vi "_s_Cambio flujos manual.vi"(7 "Comunicaciones":T2={"Flujo_1"="ASRL6::INSTR", "Brk1"=FALSE, "Flujo_2"="ASRL6::INSTR", "Brk2"=FALSE, "Flujo_3"="ASRL6::INSTR", "Brk3"=FALSE, "Flujo_4"="ASRL6::INSTR", "Brk4"=FALSE, "Eurothe"="ASRL6::INSTR", "Eurot"=FALSE, "Balanza"="ASRL6::INSTR", "Bal"=FALSE, "eValPos"="ASRL6::INSTR", "eVal"=FALSE, "flowbus"="ASRL6::INSTR", "fb"=FALSE}, 8 "error in (no error)":errorcluster, 11 "Dispositivos":T3=[["3", "NO", "M0000013", "Air", "1", "ln/mn", "0", "0"], ["4", "NO", "M0000014", "Air", "1", "ln/mn", "0", "0"], ["5", "NO", "M0000015", "Air", "1", "ln/mn", "0", "0"], ["6", "NO", "M0000016", "Air", "1", "ln/mn", "0", "0"], ["7", "NO", "M0000017", "Air", "1", "ln/mn", "0", "0"], ["8", "NO", "M0000018", "Air", "1", "ln/mn", "0", "0"], ["9", "NO", "M0000019", "Air", "1", "ln/mn", "0", "0"], ["10", "NO", "M0000020", "Air", "1", "ln/mn", "0", "0"], ["11", "NO", "M0000021", "Air", "1", "ln/mn", "0", "0"]] caption="MassFlowControllers") -> (0 "error out":errorcluster, 1 "Setpoints":T1 {"SP4" format="%.2f"; "SP3" format="%.2f"; "SP2" format="%.2f"; "SP1" format="%.2f"})   [LabVIEW 2013]
doc: "Use this template to create a dialog box. This template polls the state of the buttons on the front panel and does not use events. Use the Dialog Using Events template (not available in Base package) to create a dialog box with event handling."
uses:
  _s_TablaBronkhorst.ctl
  Controles/P2018 Com Control.ctl
  Controles/P2019 SetpointsFlows.ctl
  _s_Bronkhorst Control.ctl
panel:
  out "SP4":dbl format="%.2f"
  out "SP3":dbl format="%.2f"
  out "SP2":dbl format="%.2f"
  in  "Salir":bool
  out "SP1":dbl format="%.2f"
  in  "Add 4":bool
  in  "Add 3":bool
  in  "Add 2":bool
  in  "Add 1":bool
  # "Nuevos flujos de gases (SERIE)"
  # "Setpoint"
  # "Nota: \nAl hacer CLICK en el pulsador aparecerá\nla ventana para establecer el nuevo setpoint"
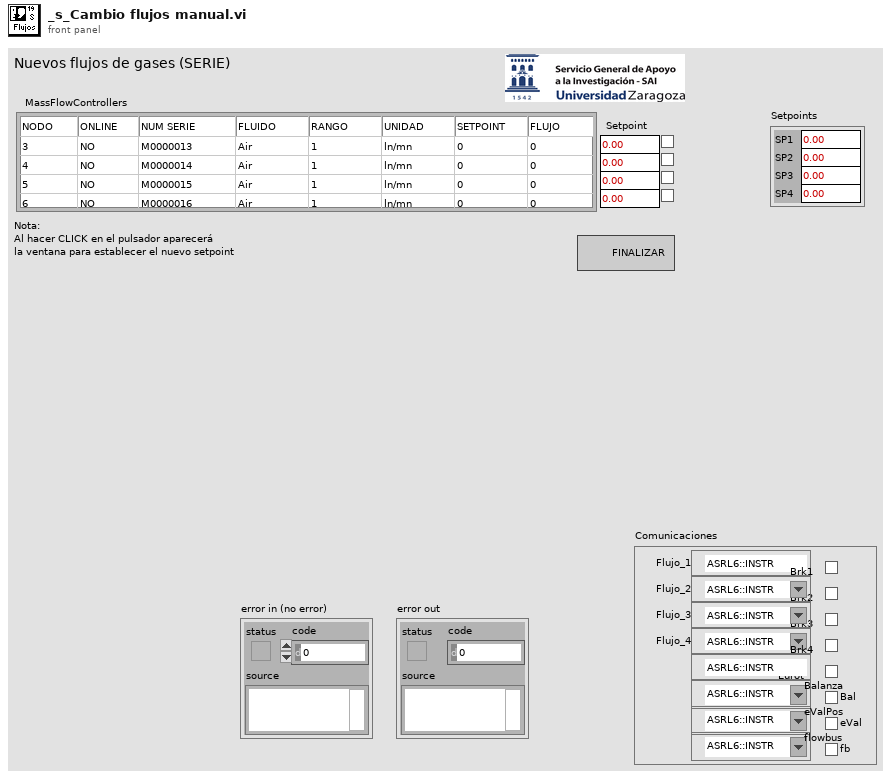
[diagram p1: front panel]
types:
  T1 = typedef "P2019 SetpointsFlows.ctl" = cluster{"SP1":dbl, "SP2":dbl, "SP3":dbl, "SP4":dbl}
  T2 = typedef "P2018 Com Control.ctl" = cluster{"Flujo_1":refnum<visa-resource-name>, "Brk1":bool, "Flujo_2":refnum<visa-resource-name>, "Brk2":bool, "Flujo_3":refnum<visa-resource-name>, "Brk3":bool, "Flujo_4":refnum<visa-resource-name>, "Brk4":bool, "Eurothe":refnum<visa-resource-name>, "Eurot":bool, "Balanza":refnum<visa-resource-name>, "Bal":bool, "eValPos":refnum<visa-resource-name>, "eVal":bool, "flowbus":refnum<visa-resource-name>, "fb":bool}
  T3 = typedef "_s_TablaBronkhorst.ctl" = string[][]
  T4 = typedef "_s_Bronkhorst Control.ctl" = enum16{"Inicializar", "Request IdnString", "Request Serial Number", "Request Fluid Number", "Request Fluid Name", "Request Sensor Type", "Request Cap 0", "Request Cap100", "Request Units", "Request CapUnitStr", "Request Setpoint %", "Request Setpoint", "Request Measure %", "Request Measure ", "Send Control Mode", "Send Fluid Number", "Send Setpoint %", "Send Setpoint", "Shutdown"}
  T5 = cluster{"SP1":dbl, "SP2":dbl, "SP3":dbl, "SP4":dbl}
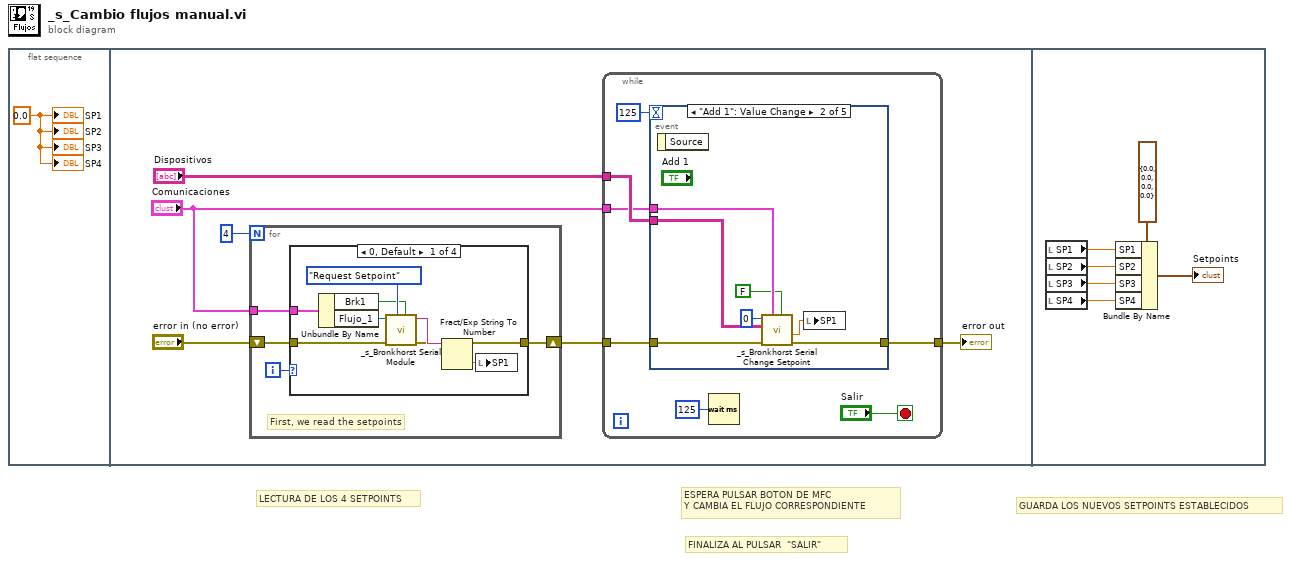
[diagram p0: block diagram]
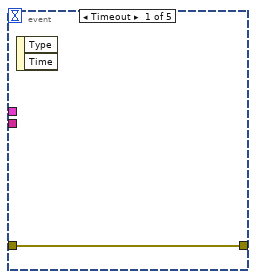
[diagram p2: hidden frame]
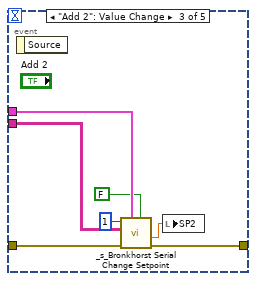
[diagram p3: hidden frame]
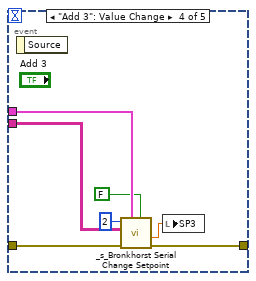
[diagram p4: hidden frame]
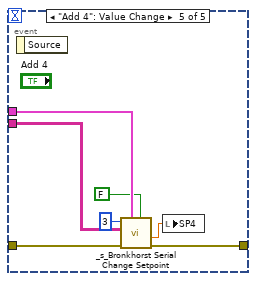
[diagram p5: hidden frame]
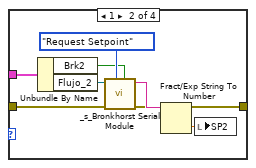
[diagram p6: hidden frame]
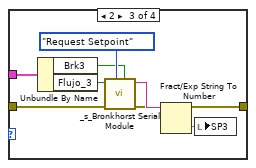
[diagram p7: hidden frame]
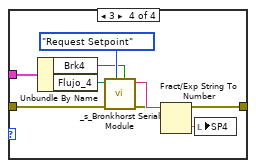
[diagram p8: hidden frame]
diagram:
  # "FINALIZA AL PULSAR  \"SALIR\""
  # "GUARDA LOS NUEVOS SETPOINTS ESTABLECIDOS"
  # "ESPERA PULSAR BOTON DE MFC\nY CAMBIA EL FLUJO CORRESPONDIENTE"
  # "LECTURA DE LOS 4 SETPOINTS"
  n1 = flat-sequence {
    frame #0 {
      w1 = 0.0 ("SP1")
      "SP1" <- w1
      "SP2" <- w1
      "SP3" <- w1
      "SP4" <- w1
    }
    frame #1 {
      n2 = for {
        N: 4 -> [_]
        shift-right: [w44] -> w5
        shift-left: "error in (no error)" -> [w45]
        tunnel: "Comunicaciones" -> [w47]
        i -> [w46]
        # "First, we read the setpoints"
        n3 = case shown="0, Default" w46 {
          tunnel: w47 -> [w55 w63 w71 w79]
          tunnel: w45 -> [w49 w57 w65 w73]
          tunnel: [w48 w56 w64 w72] -> w44
          frame 0, Default {
            n4 = Unbundle By Name(w55) -> ("Brk1"=w53:bool, "Flujo_1"=w52:refnum<visa-resource-name>)
            n5 = call "_s_Bronkhorst Serial Module.vi"("Module (T:Enable)"=w53, "Command"=_s_Bronkhorst_Control."Request Setpoint", "error in (no error)"=w49, "VISA resource name"=w52) -> ("error out"=w48:errorcluster, "Value"=w51:string)  [unwired: 4 in, 2 out]
            n6 = Fract/Exp String To Number(string=w51) -> (number=w50:dbl)  [unwired: 3 in, 1 out]
            n7 = local write "SP1"(w50) -> ()
          }
          frame 1 {
            n8 = Unbundle By Name(w63) -> ("Brk2"=w61:bool, "Flujo_2"=w60:refnum<visa-resource-name>)
            n9 = call "_s_Bronkhorst Serial Module.vi"("Module (T:Enable)"=w61, "Command"=_s_Bronkhorst_Control."Request Setpoint", "error in (no error)"=w57, "VISA resource name"=w60) -> ("error out"=w56:errorcluster, "Value"=w59:string)  [unwired: 4 in, 2 out]
            n10 = Fract/Exp String To Number(string=w59) -> (number=w58:dbl)  [unwired: 3 in, 1 out]
            n11 = local write "SP2"(w58) -> ()
          }
          frame 2 {
            n12 = Unbundle By Name(w71) -> ("Brk3"=w69:bool, "Flujo_3"=w68:refnum<visa-resource-name>)
            n13 = call "_s_Bronkhorst Serial Module.vi"("Module (T:Enable)"=w69, "Command"=_s_Bronkhorst_Control."Request Setpoint", "error in (no error)"=w65, "VISA resource name"=w68) -> ("error out"=w64:errorcluster, "Value"=w67:string)  [unwired: 4 in, 2 out]
            n14 = Fract/Exp String To Number(string=w67) -> (number=w66:dbl)  [unwired: 3 in, 1 out]
            n15 = local write "SP3"(w66) -> ()
          }
          frame 3 {
            n16 = Unbundle By Name(w79) -> ("Brk4"=w77:bool, "Flujo_4"=w76:refnum<visa-resource-name>)
            n17 = call "_s_Bronkhorst Serial Module.vi"("Module (T:Enable)"=w77, "Command"=_s_Bronkhorst_Control."Request Setpoint", "error in (no error)"=w73, "VISA resource name"=w76) -> ("error out"=w72:errorcluster, "Value"=w75:string)  [unwired: 4 in, 2 out]
            n18 = Fract/Exp String To Number(string=w75) -> (number=w74:dbl)  [unwired: 3 in, 1 out]
            n19 = local write "SP4"(w74) -> ()
          }
        }
      }
      n20 = while {
        tunnel: w5 -> [w9]
        tunnel: "Dispositivos" -> [w11]
        tunnel: "Comunicaciones" -> [w10]
        tunnel: [w8] -> w2
        stop <- "Salir" stop-if-true
        n21 = event shown="[1] \"Add 1\": Value Change" {
          selector: _ -> [_ _ _ _ _]
          dyn-events: _ -> [_ _ _ _ _]
          timeout: 125 -> [_ _ _ _ _]
          tunnel: w11 -> [_ w22 w29 w36 w43]
          tunnel: w10 -> [_ w21 w28 w35 w42]
          tunnel: w9 -> [w15 w18 w25 w32 w39]
          tunnel: [w15 w17 w24 w31 w38] -> w8
          event Timeout {
            n22 = event-data() -> ()  [unwired: 1 in, 2 out]
          }
          event "Add 1": Value Change {
            n23 = event-data() -> ()  [unwired: 1 in, 1 out]
            n24 = call "_s_Bronkhorst Serial Change Setpoint.vi"("Auto"=FALSE, "Comunicaciones"=w21, "error in (no error)"=w18, "Dispositivos"=w22, "Address"=0) -> ("error out"=w17:errorcluster, "Nuevo Setpoint 2"=w16:dbl)  [unwired: 5 in]
            n25 = local write "SP1"(w16) -> ()
          }
          event "Add 2": Value Change {
            n26 = event-data() -> ()  [unwired: 1 in, 1 out]
            n27 = call "_s_Bronkhorst Serial Change Setpoint.vi"("Auto"=FALSE, "Comunicaciones"=w28, "error in (no error)"=w25, "Dispositivos"=w29, "Address"=1) -> ("error out"=w24:errorcluster, "Nuevo Setpoint 2"=w23:dbl)  [unwired: 5 in]
            n28 = local write "SP2"(w23) -> ()
          }
          event "Add 3": Value Change {
            n29 = event-data() -> ()  [unwired: 1 in, 1 out]
            n30 = call "_s_Bronkhorst Serial Change Setpoint.vi"("Auto"=FALSE, "Comunicaciones"=w35, "error in (no error)"=w32, "Dispositivos"=w36, "Address"=2) -> ("error out"=w31:errorcluster, "Nuevo Setpoint 2"=w30:dbl)  [unwired: 5 in]
            n31 = local write "SP3"(w30) -> ()
          }
          event "Add 4": Value Change {
            n32 = event-data() -> ()  [unwired: 1 in, 1 out]
            n33 = call "_s_Bronkhorst Serial Change Setpoint.vi"("Auto"=FALSE, "Comunicaciones"=w42, "error in (no error)"=w39, "Dispositivos"=w43, "Address"=3) -> ("error out"=w38:errorcluster, "Nuevo Setpoint 2"=w37:dbl)  [unwired: 5 in]
            n34 = local write "SP4"(w37) -> ()
          }
        }
        n35 = Wait (ms)(milliseconds to wait=u32 125) -> ()  [unwired: 1 out]
      }
      "error out" <- w2
    }
    frame #2 {
      n36 = local read "SP1"() -> (w83:dbl)
      n37 = local read "SP2"() -> (w82:dbl)
      n38 = local read "SP3"() -> (w81:dbl)
      n39 = local read "SP4"() -> (w80:dbl)
      n40 = Bundle By Name(cluster=T5 {"SP1"=0.0, "SP2"=0.0, "SP3"=0.0, "SP4"=0.0} ("Setpoints"), "SP1"=w83, "SP2"=w82, "SP3"=w81, "SP4"=w80) -> (→"Setpoints":T5)
    }
  }
